vi "MGCC_FntStaMach_FSM loop.vi"() -> (0 "Function":bool[](array[boolean]), 1 "State":bool[](array[boolean]), 2 "Name of state":string[](array[string]), 3 "Name_Function":string[](array[string]), 4 "Next State":string, 5 "Current State":string)   [LabVIEW 2016]
doc: "This VI is the main loop for the FSM in MGCC. The inputs are the events while the output is the name of the next state."
uses:
  <vilib>/imath/engines/lvmath2/RunTimeEngine/IndexRead/NIMS V(S).vi
  <instcachedir>/0/NIMS V(S)_0488751826AF41519A22953C041130DC.lvgen/NIMS V(S)_0488751826AF41519A22953C041130DC_003.vi
  <vilib>/imathl/engines/lvmath/Functions/Error Handling/Create Error.vi
  <vilib>/imath/engines/lvmath2/RunTimeEngine/NodeEndStatement/NIMS_NodeEndStatement_Output.vi
  <instcachedir>/0/NIMS_NodeEndStatement_Output_53EC0D466D134D7ABD903AC30B43404B.lvgen/NIMS_NodeEndStatement_Output_53EC0D466D134D7ABD903AC30B43404B_011.vi
  <vilib>/imath/engines/lvmath2/RunTimeEngine/ErrorHandling/NIMS_Finalize Error.vi
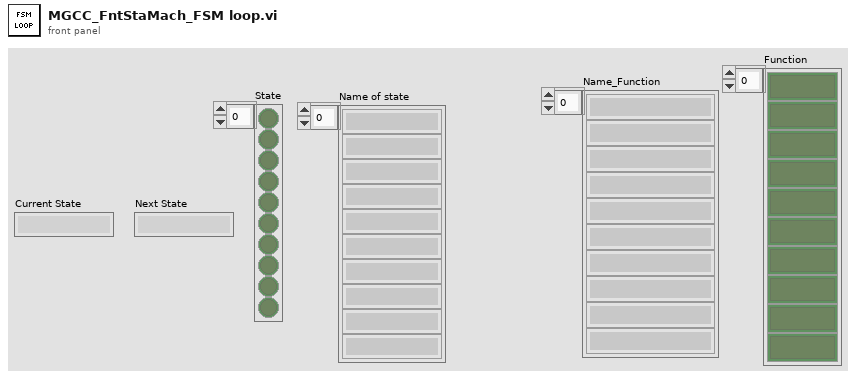
[diagram p1: front panel]
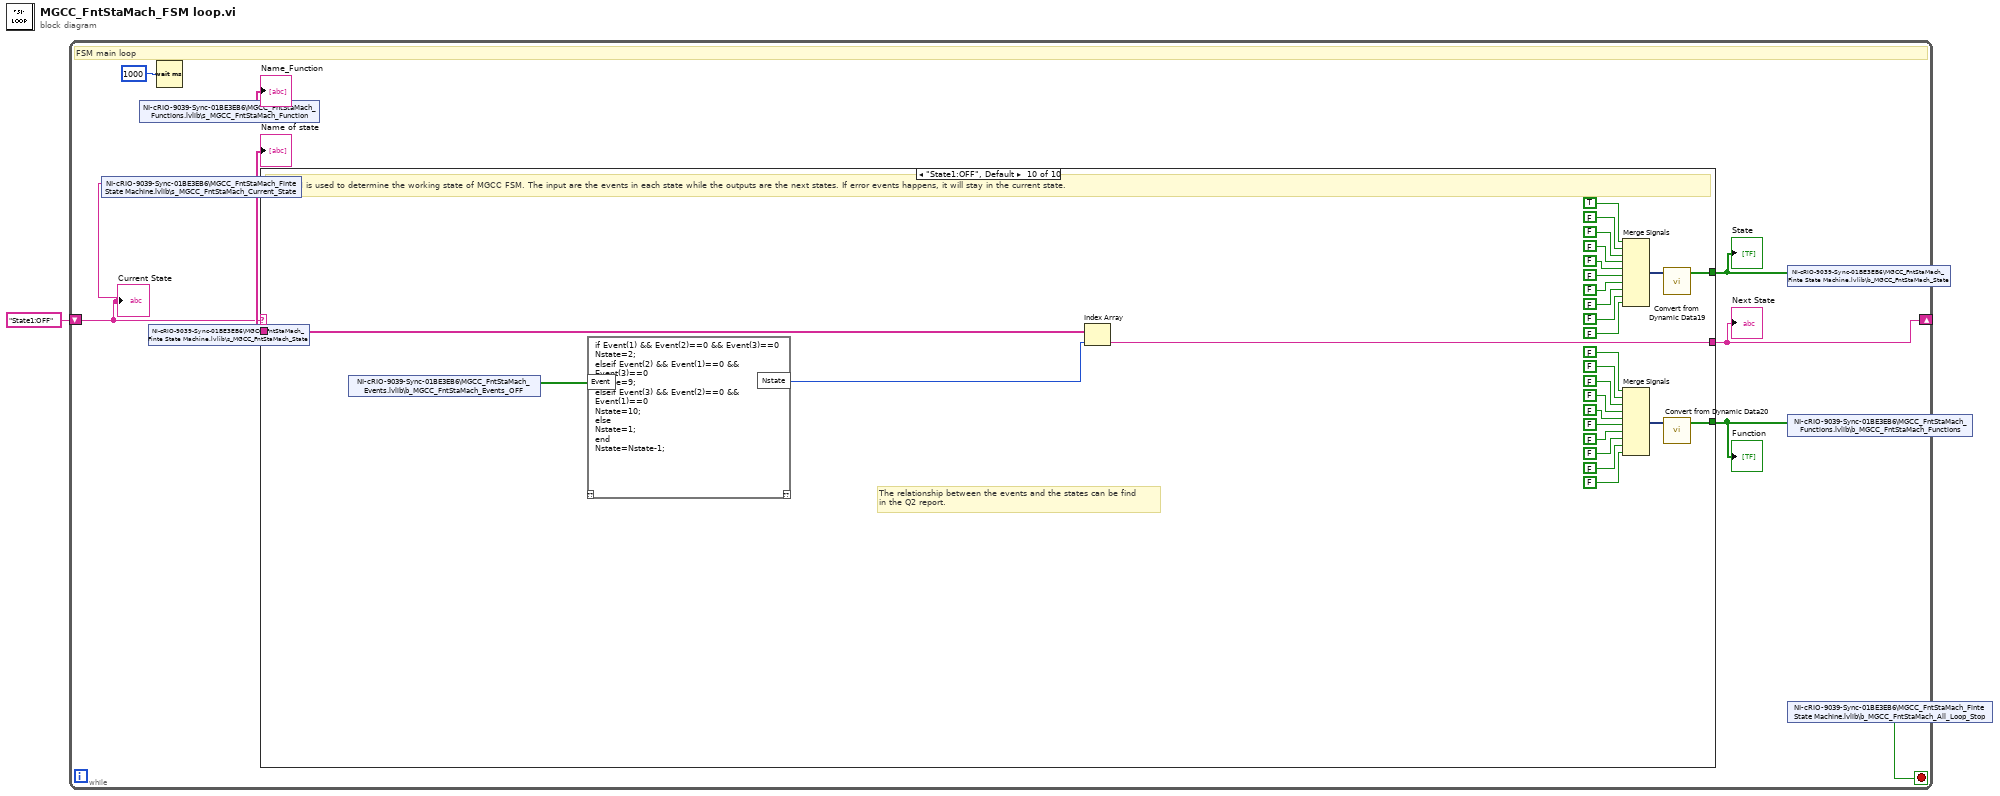
[diagram p0: block diagram]
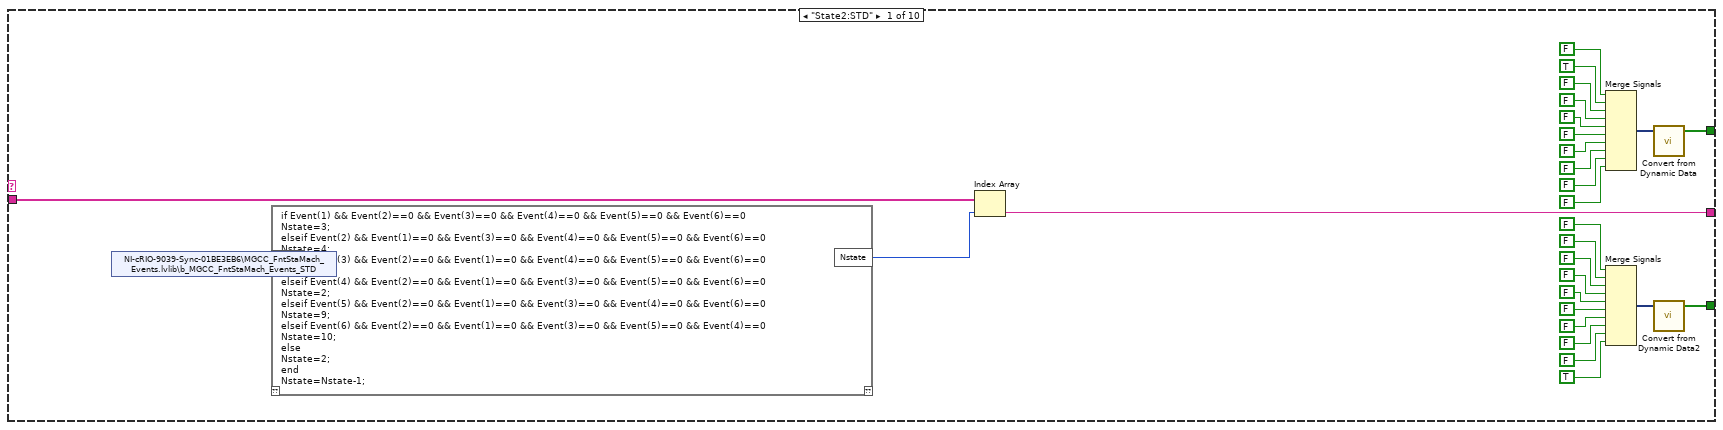
[diagram p2: hidden frame]
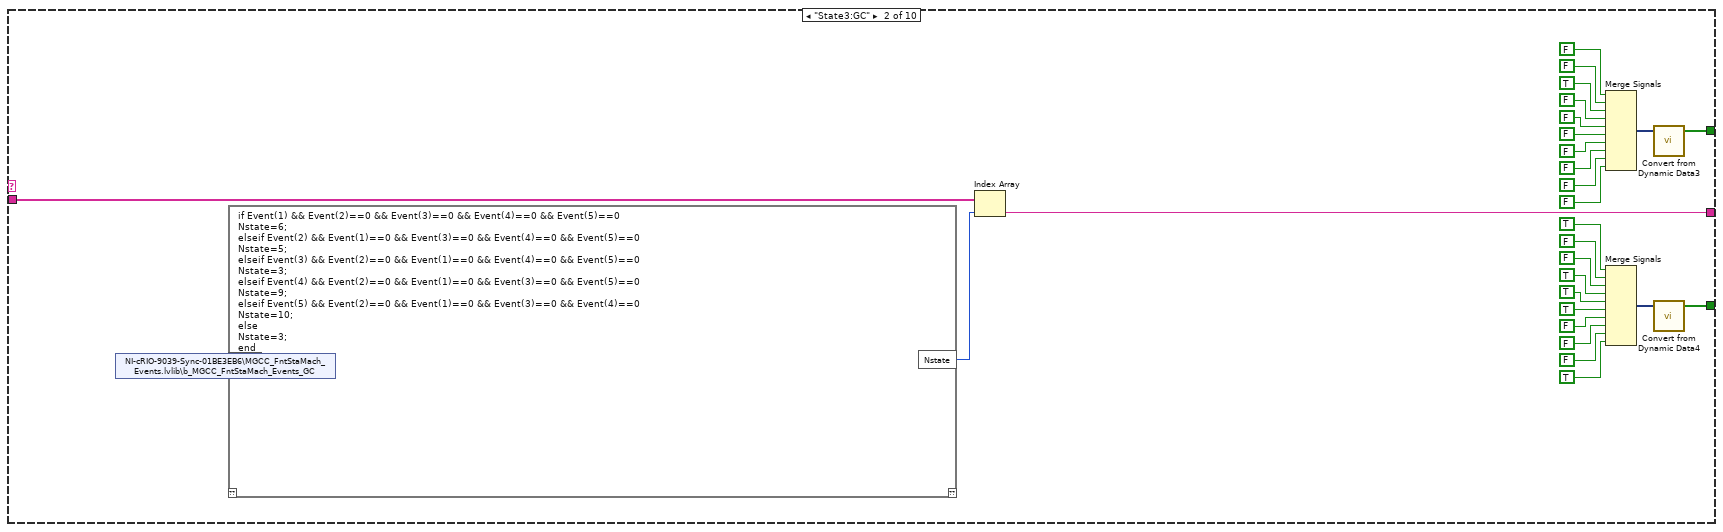
[diagram p3: hidden frame]
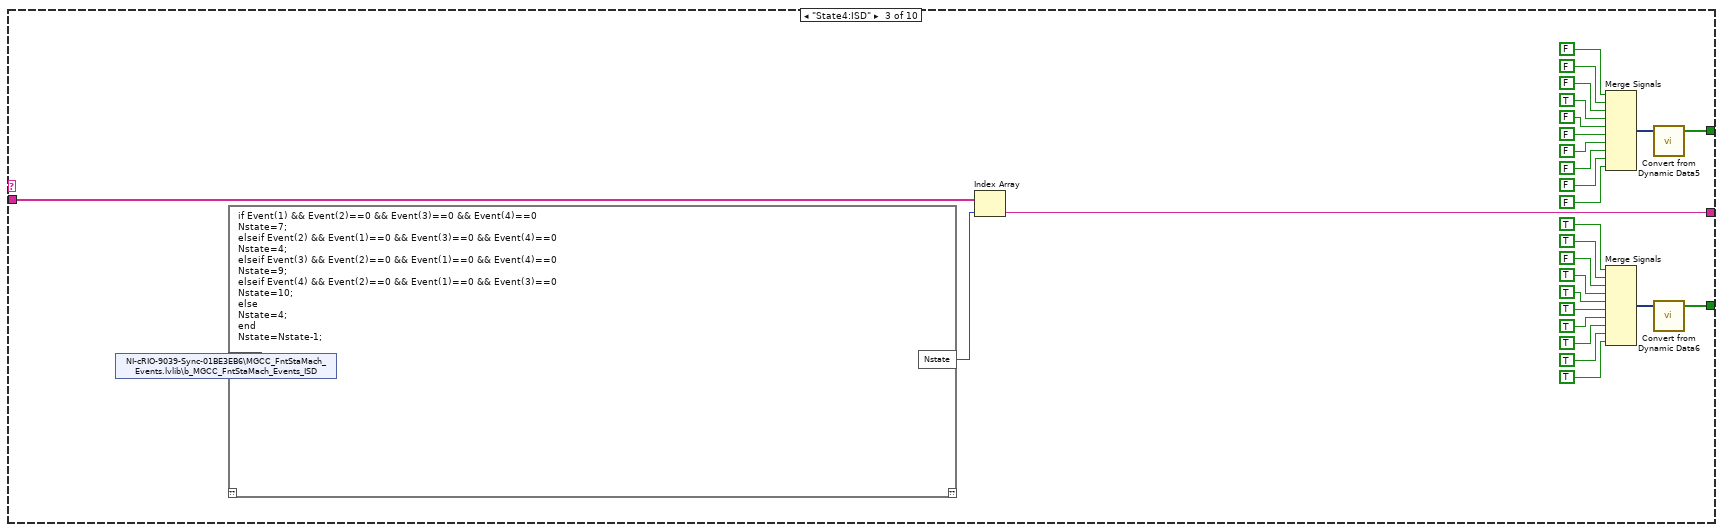
[diagram p4: hidden frame]
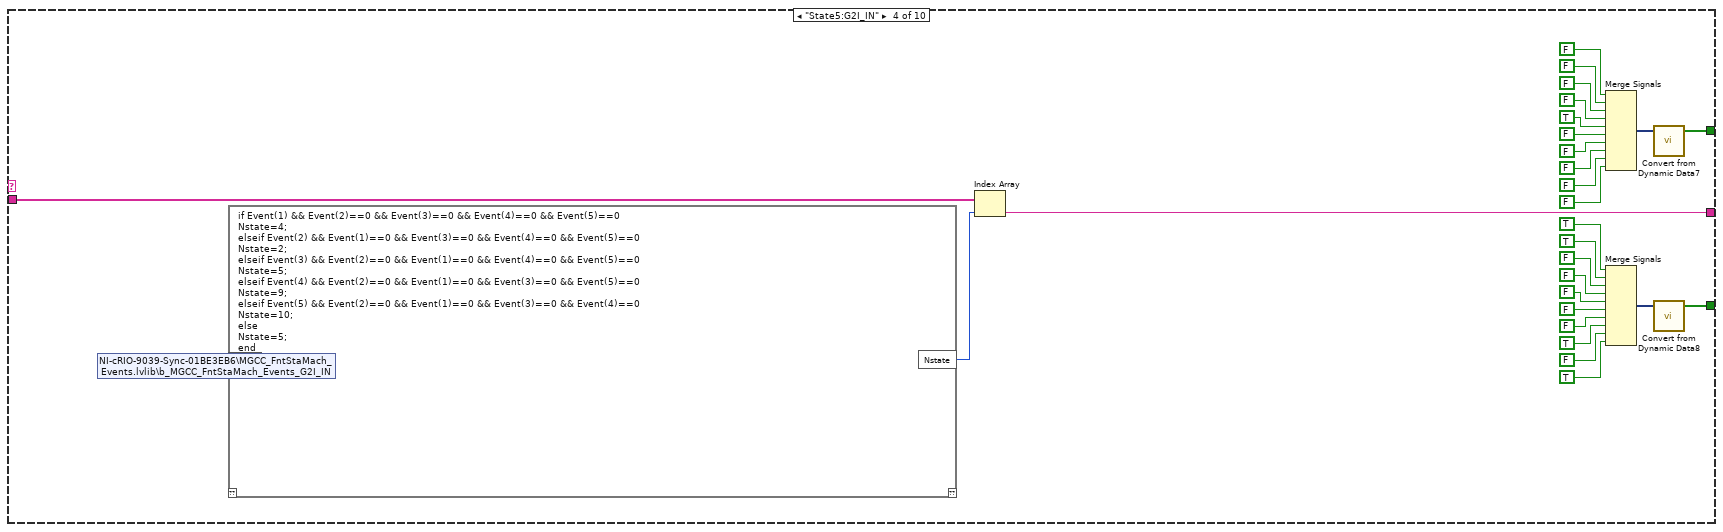
[diagram p5: hidden frame]
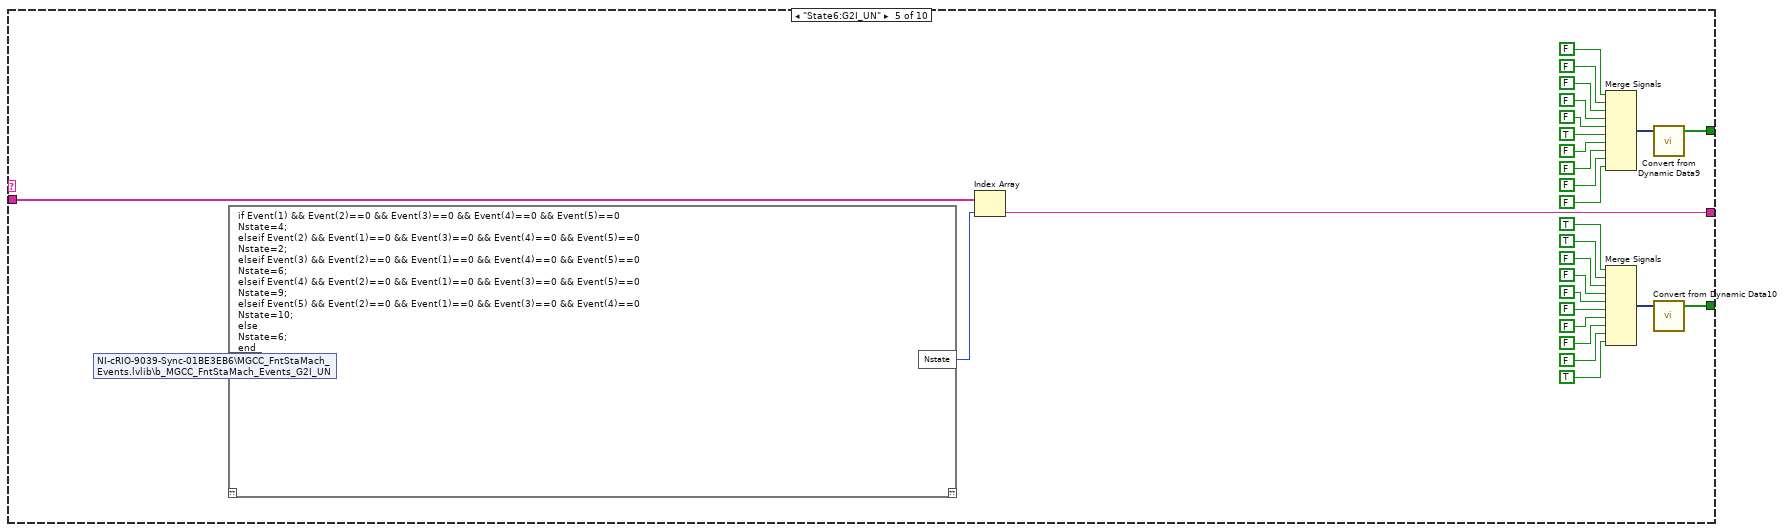
[diagram p6: hidden frame]
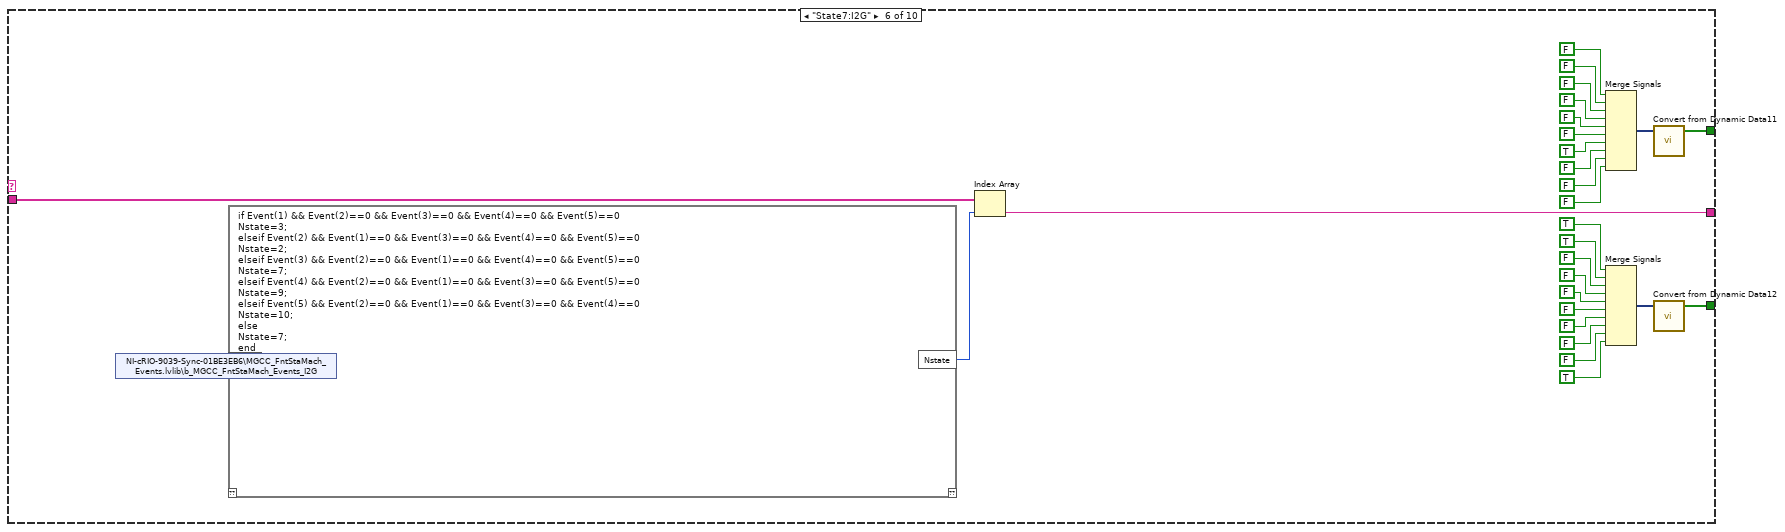
[diagram p7: hidden frame]
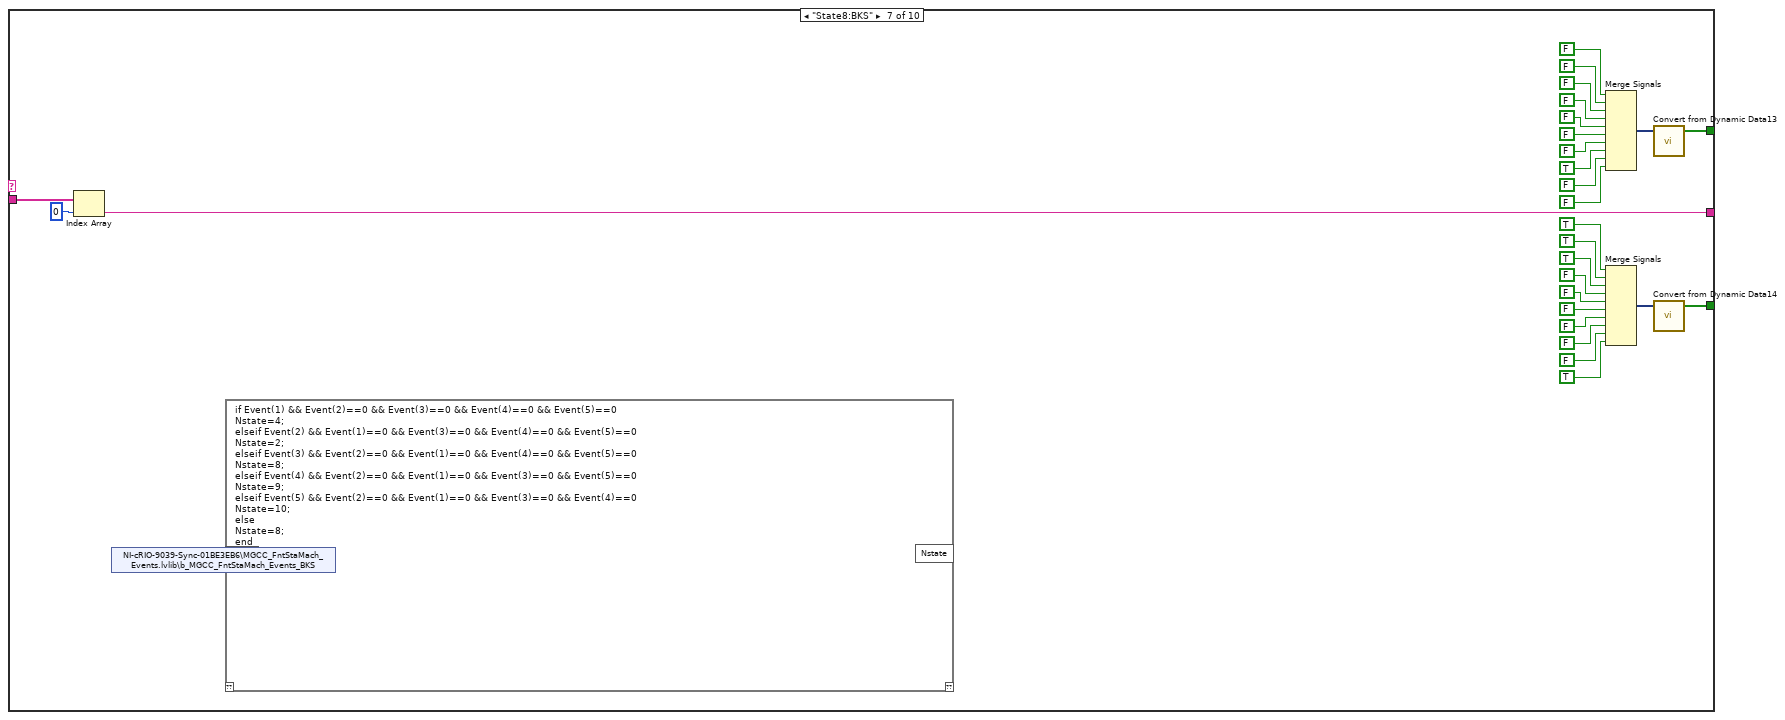
[diagram p8: hidden frame]
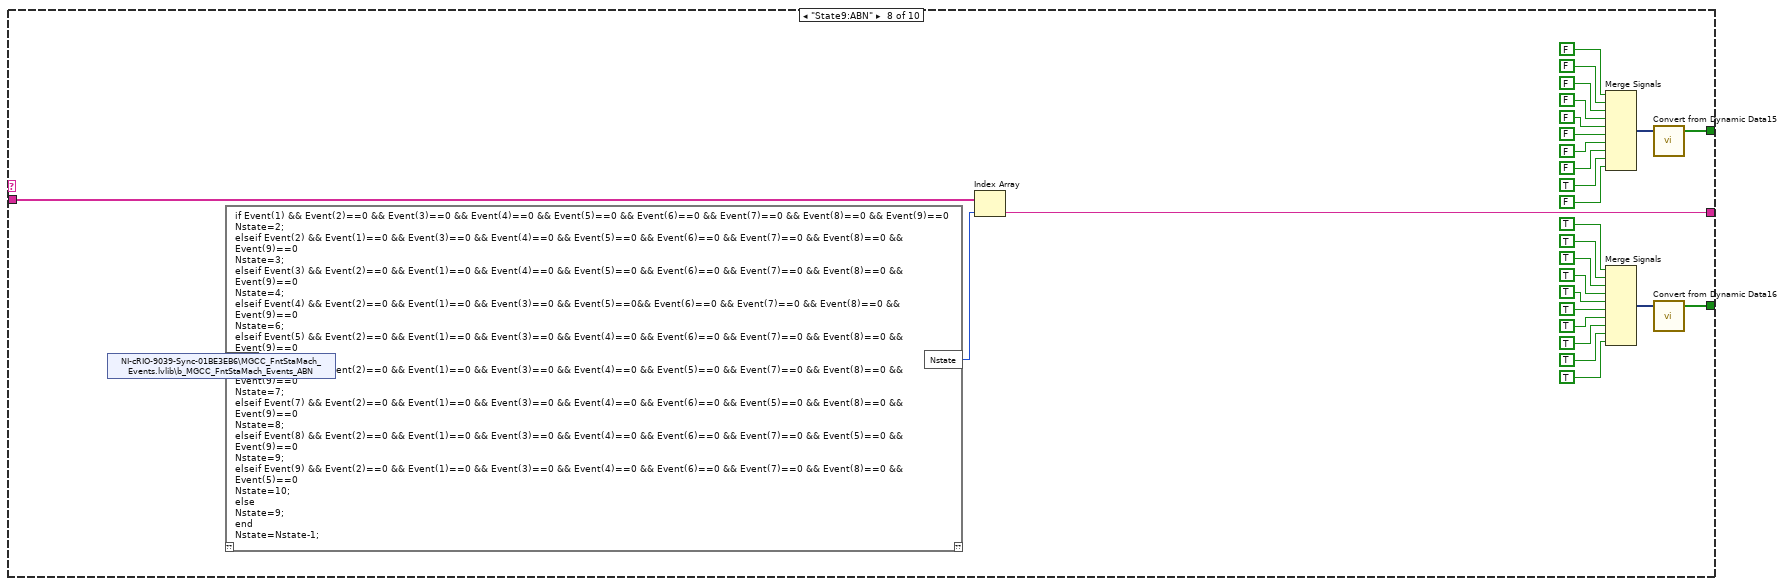
[diagram p9: hidden frame]
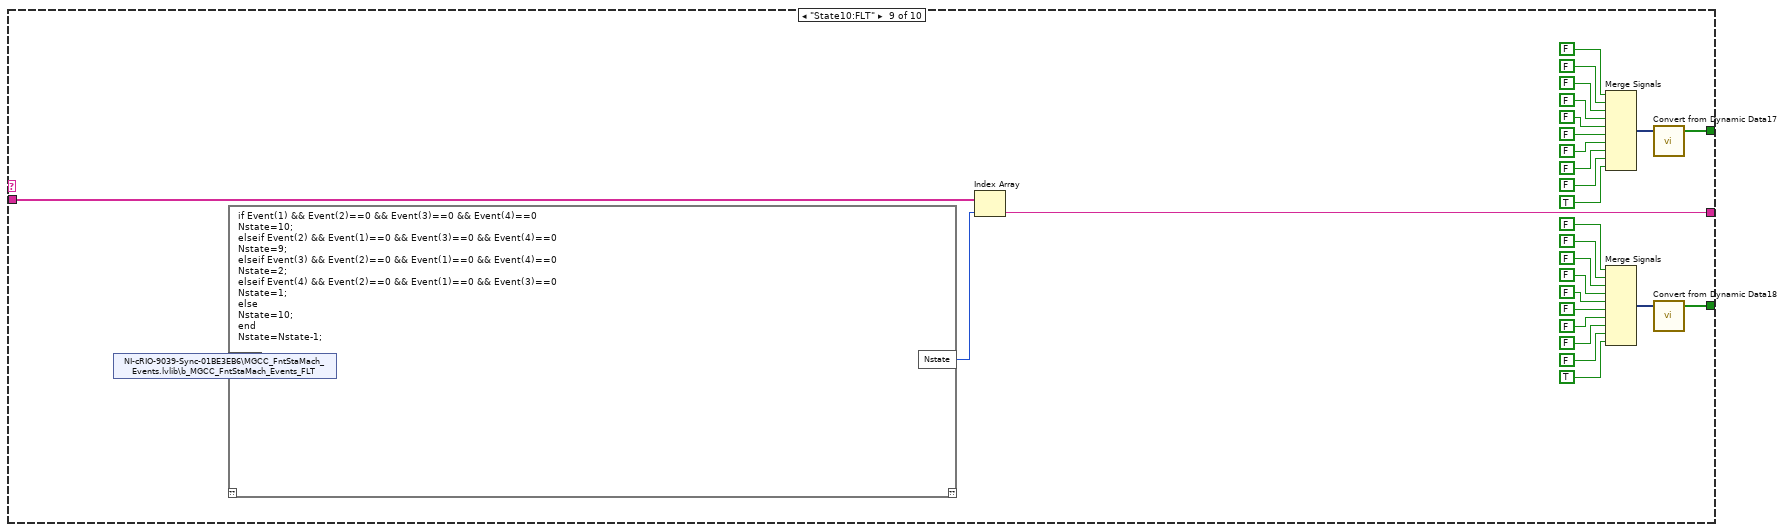
[diagram p10: hidden frame]
diagram:
  n1 = while {
    shift-right: [w9] -> _
    shift-left: "State1:OFF" ("String") -> [w2]
    stop <- w3 stop-if-true
    # "FSM main loop"
    n2 = shared-variable "NI-cRIO-9039-Sync-01BE3EB6\\MGCC_FntStaMach_Finte State Machine.lvlib\\s_MGCC_FntStaMach_Current_State"(w2) -> ()  [unwired: 1 in, 1 out]
    n3 = shared-variable "NI-cRIO-9039-Sync-01BE3EB6\\MGCC_FntStaMach_Functions.lvlib\\s_MGCC_FntStaMach_Function"() -> (→"Name_Function":string[])  [unwired: 1 in, 1 out]
    n4 = shared-variable "NI-cRIO-9039-Sync-01BE3EB6\\MGCC_FntStaMach_Finte State Machine.lvlib\\s_MGCC_FntStaMach_State"() -> (w7:string[])  [unwired: 1 in, 1 out]
    "Name of state" <- w7
    n5 = Wait (ms)(milliseconds to wait=u32 1000) -> ()  [unwired: 1 out]
    n6 = case shown="\"State1:OFF\", Default" w2 {
      tunnel: [w37 w1004 w1703 w2172 w2871 w3570 w4268 w4968 w7087 w7568] -> w9
      tunnel: [w25 w1005 w1704 w2173 w2872 w3571 w4270 w4969 w7088 w7556] -> w6
      tunnel: w7 -> [w24 w1003 w1702 w2171 w2870 w3569 w4267 w4967 w7086 w7555]
      tunnel: [w10 w989 w1688 w2157 w2856 w3555 w4254 w4953 w7072 w7541] -> w5
      frame "State2:STD" {
        n7 = shared-variable "NI-cRIO-9039-Sync-01BE3EB6\\MGCC_FntStaMach_Events.lvlib\\b_MGCC_FntStaMach_Events_STD"() -> (w23:bool[])  [unwired: 1 in, 1 out]
        n8 = mathscript code="if Event(1) && Event(2)==0 && Event(3)==0 && Event(4)==0 && Event(5)==0 && Event(6)==0\nNstate=3;\nelseif Event(2) && Event(1)==0 && Event(3)==0 && Event(4)==0 && Event(5)==0 && Event(6)==0\nNstate=4;\nelseif Event(3) && Event(2)==0 && Event(1)==0 && Event(4)==0 && Event(5)==0 && Event(6)==0\nNstate=8;\nelseif Event(4) && Event(2)==0 && Event(1)==0 && Event(3)==0 && Event(5)==0 && Event(6)==0\nNstate=2;\nelseif Event(5) && Event(2)==0 && Event(1)==0 && Event(3)==0 && Event(4)==0 && Event(6)==0\nNstate=9;\nelseif Event(6) && Event(2)==0 && Event(1)==0 && Event(3)==0 && Event(5)==0 && Event(4)==0\nNstate=10;\nelse\nNstate=2;\nend\nNstate=Nstate-1;"("Event"=w23) -> ("Nstate"=w22:i32)  [unwired: 1 in, 1 out]
        n9 = Index Array(array=w24, index=w22) -> (element=w37:string)
        n10 = Merge Signals(FALSE ("State3"), TRUE ("State3"), FALSE ("State3"), FALSE ("State3"), FALSE ("State3"), FALSE ("State3"), FALSE ("State3"), FALSE ("State3"), FALSE ("State3"), FALSE ("State3")) -> (w26:dynamicdata)
        n11 = Merge Signals(FALSE ("State3"), FALSE ("State3"), FALSE ("State3"), FALSE ("State3"), FALSE ("State3"), FALSE ("State3"), FALSE ("State3"), FALSE ("State3"), FALSE ("State3"), TRUE ("State3")) -> (w11:dynamicdata)
        n12 = call "Convert from Dynamic Data"("Dynamic Data Type"=w26) -> ("Array"=w25:bool[])  [unwired: 3 in]
        n13 = call "Convert from Dynamic Data2"("Dynamic Data Type"=w11) -> ("Array"=w10:bool[])  [unwired: 3 in]
      }
      frame "State3:GC" {
        n14 = shared-variable "NI-cRIO-9039-Sync-01BE3EB6\\MGCC_FntStaMach_Events.lvlib\\b_MGCC_FntStaMach_Events_GC"() -> (w1002:bool[])  [unwired: 1 in, 1 out]
        n15 = mathscript code="if Event(1) && Event(2)==0 && Event(3)==0 && Event(4)==0 && Event(5)==0 \nNstate=6;\nelseif Event(2) && Event(1)==0 && Event(3)==0 && Event(4)==0 && Event(5)==0 \nNstate=5;\nelseif Event(3) && Event(2)==0 && Event(1)==0 && Event(4)==0 && Event(5)==0 \nNstate=3;\nelseif Event(4) && Event(2)==0 && Event(1)==0 && Event(3)==0 && Event(5)==0\nNstate=9;\nelseif Event(5) && Event(2)==0 && Event(1)==0 && Event(3)==0 && Event(4)==0 \nNstate=10;\nelse\nNstate=3;\nend\nNstate=Nstate-1;"("Event"=w1002) -> ("Nstate"=w1001:i32)  [unwired: 1 in, 1 out]
        n16 = Index Array(array=w1003, index=w1001) -> (element=w1004:string)
        n17 = Merge Signals(FALSE ("State3"), FALSE ("State3"), TRUE ("State3"), FALSE ("State3"), FALSE ("State3"), FALSE ("State3"), FALSE ("State3"), FALSE ("State3"), FALSE ("State3"), FALSE ("State3")) -> (w1006:dynamicdata)
        n18 = Merge Signals(TRUE ("State3"), FALSE ("State3"), FALSE ("State3"), TRUE ("State3"), TRUE ("State3"), TRUE ("State3"), FALSE ("State3"), FALSE ("State3"), FALSE ("State3"), TRUE ("State3")) -> (w990:dynamicdata)
        n19 = call "Convert from Dynamic Data3"("Dynamic Data Type"=w1006) -> ("Array"=w1005:bool[])  [unwired: 3 in]
        n20 = call "Convert from Dynamic Data4"("Dynamic Data Type"=w990) -> ("Array"=w989:bool[])  [unwired: 3 in]
      }
      frame "State4:ISD" {
        n21 = shared-variable "NI-cRIO-9039-Sync-01BE3EB6\\MGCC_FntStaMach_Events.lvlib\\b_MGCC_FntStaMach_Events_ISD"() -> (w1701:bool[])  [unwired: 1 in, 1 out]
        n22 = mathscript code="if Event(1) && Event(2)==0 && Event(3)==0 && Event(4)==0 \nNstate=7;\nelseif Event(2) && Event(1)==0 && Event(3)==0 && Event(4)==0 \nNstate=4;\nelseif Event(3) && Event(2)==0 && Event(1)==0 && Event(4)==0 \nNstate=9;\nelseif Event(4) && Event(2)==0 && Event(1)==0 && Event(3)==0 \nNstate=10;\nelse\nNstate=4;\nend\nNstate=Nstate-1;"("Event"=w1701) -> ("Nstate"=w1700:i32)  [unwired: 1 in, 1 out]
        n23 = Index Array(array=w1702, index=w1700) -> (element=w1703:string)
        n24 = Merge Signals(FALSE ("State3"), FALSE ("State3"), FALSE ("State3"), TRUE ("State3"), FALSE ("State3"), FALSE ("State3"), FALSE ("State3"), FALSE ("State3"), FALSE ("State3"), FALSE ("State3")) -> (w1705:dynamicdata)
        n25 = Merge Signals(TRUE ("State3"), TRUE ("State3"), FALSE ("State3"), TRUE ("State3"), TRUE ("State3"), TRUE ("State3"), TRUE ("State3"), TRUE ("State3"), TRUE ("State3"), TRUE ("State3")) -> (w1689:dynamicdata)
        n26 = call "Convert from Dynamic Data5"("Dynamic Data Type"=w1705) -> ("Array"=w1704:bool[])  [unwired: 3 in]
        n27 = call "Convert from Dynamic Data6"("Dynamic Data Type"=w1689) -> ("Array"=w1688:bool[])  [unwired: 3 in]
      }
      frame "State5:G2I_IN" {
        n28 = shared-variable "NI-cRIO-9039-Sync-01BE3EB6\\MGCC_FntStaMach_Events.lvlib\\b_MGCC_FntStaMach_Events_G2I_IN"() -> (w2170:bool[])  [unwired: 1 in, 1 out]
        n29 = mathscript code="if Event(1) && Event(2)==0 && Event(3)==0 && Event(4)==0 && Event(5)==0 \nNstate=4;\nelseif Event(2) && Event(1)==0 && Event(3)==0 && Event(4)==0 && Event(5)==0 \nNstate=2;\nelseif Event(3) && Event(2)==0 && Event(1)==0 && Event(4)==0 && Event(5)==0 \nNstate=5;\nelseif Event(4) && Event(2)==0 && Event(1)==0 && Event(3)==0 && Event(5)==0\nNstate=9;\nelseif Event(5) && Event(2)==0 && Event(1)==0 && Event(3)==0 && Event(4)==0 \nNstate=10;\nelse\nNstate=5;\nend\nNstate=Nstate-1;"("Event"=w2170) -> ("Nstate"=w2169:i32)  [unwired: 1 in, 1 out]
        n30 = Index Array(array=w2171, index=w2169) -> (element=w2172:string)
        n31 = Merge Signals(FALSE ("State3"), FALSE ("State3"), FALSE ("State3"), FALSE ("State3"), TRUE ("State3"), FALSE ("State3"), FALSE ("State3"), FALSE ("State3"), FALSE ("State3"), FALSE ("State3")) -> (w2174:dynamicdata)
        n32 = Merge Signals(TRUE ("State3"), TRUE ("State3"), FALSE ("State3"), FALSE ("State3"), FALSE ("State3"), FALSE ("State3"), FALSE ("State3"), TRUE ("State3"), FALSE ("State3"), TRUE ("State3")) -> (w2158:dynamicdata)
        n33 = call "Convert from Dynamic Data7"("Dynamic Data Type"=w2174) -> ("Array"=w2173:bool[])  [unwired: 3 in]
        n34 = call "Convert from Dynamic Data8"("Dynamic Data Type"=w2158) -> ("Array"=w2157:bool[])  [unwired: 3 in]
      }
      frame "State6:G2I_UN" {
        n35 = shared-variable "NI-cRIO-9039-Sync-01BE3EB6\\MGCC_FntStaMach_Events.lvlib\\b_MGCC_FntStaMach_Events_G2I_UN"() -> (w2868:bool[])  [unwired: 1 in, 1 out]
        n36 = mathscript code="if Event(1) && Event(2)==0 && Event(3)==0 && Event(4)==0 && Event(5)==0 \nNstate=4;\nelseif Event(2) && Event(1)==0 && Event(3)==0 && Event(4)==0 && Event(5)==0 \nNstate=2;\nelseif Event(3) && Event(2)==0 && Event(1)==0 && Event(4)==0 && Event(5)==0 \nNstate=6;\nelseif Event(4) && Event(2)==0 && Event(1)==0 && Event(3)==0 && Event(5)==0\nNstate=9;\nelseif Event(5) && Event(2)==0 && Event(1)==0 && Event(3)==0 && Event(4)==0 \nNstate=10;\nelse\nNstate=6;\nend\nNstate=Nstate-1;"("Event"=w2868) -> ("Nstate"=w2869:i32)  [unwired: 1 in, 1 out]
        n37 = Index Array(array=w2870, index=w2869) -> (element=w2871:string)
        n38 = Merge Signals(FALSE ("State3"), FALSE ("State3"), FALSE ("State3"), FALSE ("State3"), FALSE ("State3"), TRUE ("State3"), FALSE ("State3"), FALSE ("State3"), FALSE ("State3"), FALSE ("State3")) -> (w2873:dynamicdata)
        n39 = Merge Signals(TRUE ("State3"), TRUE ("State3"), FALSE ("State3"), FALSE ("State3"), FALSE ("State3"), FALSE ("State3"), FALSE ("State3"), FALSE ("State3"), FALSE ("State3"), TRUE ("State3")) -> (w2857:dynamicdata)
        n40 = call "Convert from Dynamic Data9"("Dynamic Data Type"=w2873) -> ("Array"=w2872:bool[])  [unwired: 3 in]
        n41 = call "Convert from Dynamic Data10"("Dynamic Data Type"=w2857) -> ("Array"=w2856:bool[])  [unwired: 3 in]
      }
      frame "State7:I2G" {
        n42 = shared-variable "NI-cRIO-9039-Sync-01BE3EB6\\MGCC_FntStaMach_Events.lvlib\\b_MGCC_FntStaMach_Events_I2G"() -> (w3567:bool[])  [unwired: 1 in, 1 out]
        n43 = mathscript code="if Event(1) && Event(2)==0 && Event(3)==0 && Event(4)==0 && Event(5)==0 \nNstate=3;\nelseif Event(2) && Event(1)==0 && Event(3)==0 && Event(4)==0 && Event(5)==0 \nNstate=2;\nelseif Event(3) && Event(2)==0 && Event(1)==0 && Event(4)==0 && Event(5)==0 \nNstate=7;\nelseif Event(4) && Event(2)==0 && Event(1)==0 && Event(3)==0 && Event(5)==0\nNstate=9;\nelseif Event(5) && Event(2)==0 && Event(1)==0 && Event(3)==0 && Event(4)==0 \nNstate=10;\nelse\nNstate=7;\nend\nNstate=Nstate-1;"("Event"=w3567) -> ("Nstate"=w3568:i32)  [unwired: 1 in, 1 out]
        n44 = Index Array(array=w3569, index=w3568) -> (element=w3570:string)
        n45 = Merge Signals(FALSE ("State3"), FALSE ("State3"), FALSE ("State3"), FALSE ("State3"), FALSE ("State3"), FALSE ("State3"), TRUE ("State3"), FALSE ("State3"), FALSE ("State3"), FALSE ("State3")) -> (w3572:dynamicdata)
        n46 = Merge Signals(TRUE ("State3"), TRUE ("State3"), FALSE ("State3"), FALSE ("State3"), FALSE ("State3"), FALSE ("State3"), FALSE ("State3"), FALSE ("State3"), FALSE ("State3"), TRUE ("State3")) -> (w3556:dynamicdata)
        n47 = call "Convert from Dynamic Data11"("Dynamic Data Type"=w3572) -> ("Array"=w3571:bool[])  [unwired: 3 in]
        n48 = call "Convert from Dynamic Data12"("Dynamic Data Type"=w3556) -> ("Array"=w3555:bool[])  [unwired: 3 in]
      }
      frame "State8:BKS" {
        n49 = Index Array(array=w4267, index=0) -> (element=w4268:string)
        n50 = shared-variable "NI-cRIO-9039-Sync-01BE3EB6\\MGCC_FntStaMach_Events.lvlib\\b_MGCC_FntStaMach_Events_BKS"() -> (w4266:bool[])  [unwired: 1 in, 1 out]
        n51 = mathscript code="if Event(1) && Event(2)==0 && Event(3)==0 && Event(4)==0 && Event(5)==0 \nNstate=4;\nelseif Event(2) && Event(1)==0 && Event(3)==0 && Event(4)==0 && Event(5)==0 \nNstate=2;\nelseif Event(3) && Event(2)==0 && Event(1)==0 && Event(4)==0 && Event(5)==0 \nNstate=8;\nelseif Event(4) && Event(2)==0 && Event(1)==0 && Event(3)==0 && Event(5)==0\nNstate=9;\nelseif Event(5) && Event(2)==0 && Event(1)==0 && Event(3)==0 && Event(4)==0 \nNstate=10;\nelse\nNstate=8;\nend\nNstate=Nstate-1;"("Event"=w4266) -> ()  [unwired: 1 in, 2 out]
        n52 = Merge Signals(FALSE ("State3"), FALSE ("State3"), FALSE ("State3"), FALSE ("State3"), FALSE ("State3"), FALSE ("State3"), FALSE ("State3"), TRUE ("State3"), FALSE ("State3"), FALSE ("State3")) -> (w4271:dynamicdata)
        n53 = Merge Signals(TRUE ("State3"), TRUE ("State3"), TRUE ("State3"), FALSE ("State3"), FALSE ("State3"), FALSE ("State3"), FALSE ("State3"), FALSE ("State3"), FALSE ("State3"), TRUE ("State3")) -> (w4255:dynamicdata)
        n54 = call "Convert from Dynamic Data13"("Dynamic Data Type"=w4271) -> ("Array"=w4270:bool[])  [unwired: 3 in]
        n55 = call "Convert from Dynamic Data14"("Dynamic Data Type"=w4255) -> ("Array"=w4254:bool[])  [unwired: 3 in]
      }
      frame "State9:ABN" {
        n56 = shared-variable "NI-cRIO-9039-Sync-01BE3EB6\\MGCC_FntStaMach_Events.lvlib\\b_MGCC_FntStaMach_Events_ABN"() -> (w4966:bool[])  [unwired: 1 in, 1 out]
        n57 = mathscript code="if Event(1) && Event(2)==0 && Event(3)==0 && Event(4)==0 && Event(5)==0 && Event(6)==0 && Event(7)==0 && Event(8)==0 && Event(9)==0 \nNstate=2;\nelseif Event(2) && Event(1)==0 && Event(3)==0 && Event(4)==0 && Event(5)==0 && Event(6)==0 && Event(7)==0 && Event(8)==0 && Event(9)==0 \nNstate=3;\nelseif Event(3) && Event(2)==0 && Event(1)==0 && Event(4)==0 && Event(5)==0 && Event(6)==0 && Event(7)==0 && Event(8)==0 && Event(9)==0 \nNstate=4;\nelseif Event(4) && Event(2)==0 && Event(1)==0 && Event(3)==0 && Event(5)==0&& Event(6)==0 && Event(7)==0 && Event(8)==0 && Event(9)==0 \nNstate=6;\nelseif Event(5) && Event(2)==0 && Event(1)==0 && Event(3)==0 && Event(4)==0 && Event(6)==0 && Event(7)==0 && Event(8)==0 && Event(9)==0 \nNstate=5;\nelseif Event(6) && Event(2)==0 && Event(1)==0 && Event(3)==0 && Event(4)==0 && Event(5)==0 && Event(7)==0 && Event(8)==0 && Event(9)==0 \nNstate=7;\nelseif Event(7) && Event(2)==0 && Event(1)==0 && Event(3)==0 && Event(4)==0 && Event(6)==0 && Event(5)==0 && Event(8)==0 && Event(9)==0 \nNstate=8;\nelseif Event(8) && Event(2)==0 && Event(1)==0 && Event(3)==0 && Event(4)==0 && Event(6)==0 && Event(7)==0 && Event(5)==0 && Event(9)==0 \nNstate=9;\nelseif Event(9) && Event(2)==0 && Event(1)==0 && Event(3)==0 && Event(4)==0 && Event(6)==0 && Event(7)==0 && Event(8)==0 && Event(5)==0 \nNstate=10;\nelse\nNstate=9;\nend\nNstate=Nstate-1;"("Event"=w4966) -> ("Nstate"=w4965:i32)  [unwired: 1 in, 1 out]
        n58 = Index Array(array=w4967, index=w4965) -> (element=w4968:string)
        n59 = Merge Signals(FALSE ("State3"), FALSE ("State3"), FALSE ("State3"), FALSE ("State3"), FALSE ("State3"), FALSE ("State3"), FALSE ("State3"), FALSE ("State3"), TRUE ("State3"), FALSE ("State3")) -> (w4970:dynamicdata)
        n60 = Merge Signals(TRUE ("State3"), TRUE ("State3"), TRUE ("State3"), TRUE ("State3"), TRUE ("State3"), TRUE ("State3"), TRUE ("State3"), TRUE ("State3"), TRUE ("State3"), TRUE ("State3")) -> (w4954:dynamicdata)
        n61 = call "Convert from Dynamic Data15"("Dynamic Data Type"=w4970) -> ("Array"=w4969:bool[])  [unwired: 3 in]
        n62 = call "Convert from Dynamic Data16"("Dynamic Data Type"=w4954) -> ("Array"=w4953:bool[])  [unwired: 3 in]
      }
      frame "State10:FLT" {
        n63 = shared-variable "NI-cRIO-9039-Sync-01BE3EB6\\MGCC_FntStaMach_Events.lvlib\\b_MGCC_FntStaMach_Events_FLT"() -> (w7085:bool[])  [unwired: 1 in, 1 out]
        n64 = mathscript code="if Event(1) && Event(2)==0 && Event(3)==0 && Event(4)==0 \nNstate=10;\nelseif Event(2) && Event(1)==0 && Event(3)==0 && Event(4)==0 \nNstate=9;\nelseif Event(3) && Event(2)==0 && Event(1)==0 && Event(4)==0 \nNstate=2;\nelseif Event(4) && Event(2)==0 && Event(1)==0 && Event(3)==0 \nNstate=1;\nelse\nNstate=10;\nend\nNstate=Nstate-1;"("Event"=w7085) -> ("Nstate"=w7084:i32)  [unwired: 1 in, 1 out]
        n65 = Index Array(array=w7086, index=w7084) -> (element=w7087:string)
        n66 = Merge Signals(FALSE ("State3"), FALSE ("State3"), FALSE ("State3"), FALSE ("State3"), FALSE ("State3"), FALSE ("State3"), FALSE ("State3"), FALSE ("State3"), FALSE ("State3"), TRUE ("State3")) -> (w7089:dynamicdata)
        n67 = Merge Signals(FALSE ("State3"), FALSE ("State3"), FALSE ("State3"), FALSE ("State3"), FALSE ("State3"), FALSE ("State3"), FALSE ("State3"), FALSE ("State3"), FALSE ("State3"), TRUE ("State3")) -> (w7073:dynamicdata)
        n68 = call "Convert from Dynamic Data17"("Dynamic Data Type"=w7089) -> ("Array"=w7088:bool[])  [unwired: 3 in]
        n69 = call "Convert from Dynamic Data18"("Dynamic Data Type"=w7073) -> ("Array"=w7072:bool[])  [unwired: 3 in]
      }
      frame "State1:OFF", Default {
        # "The relationship between the events and the states can be find\nin the Q2 report."
        # "This FSM is used to determine the working state of MGCC FSM. The input are the events in each state while the outputs are the next states. If error events happens, it will stay in the current state."
        n70 = shared-variable "NI-cRIO-9039-Sync-01BE3EB6\\MGCC_FntStaMach_Events.lvlib\\b_MGCC_FntStaMach_Events_OFF"() -> (w7554:bool[])  [unwired: 1 in, 1 out]
        n71 = mathscript code="if Event(1) && Event(2)==0 && Event(3)==0\nNstate=2;\nelseif Event(2) && Event(1)==0 && Event(3)==0\nNstate=9;\nelseif Event(3) && Event(2)==0 && Event(1)==0\nNstate=10;\nelse\nNstate=1;\nend\nNstate=Nstate-1;"("Event"=w7554) -> ("Nstate"=w7553:i32)  [unwired: 1 in, 1 out]
        n72 = Index Array(array=w7555, index=w7553) -> (element=w7568:string)
        n73 = Merge Signals(TRUE ("State3"), FALSE ("State3"), FALSE ("State3"), FALSE ("State3"), FALSE ("State3"), FALSE ("State3"), FALSE ("State3"), FALSE ("State3"), FALSE ("State3"), FALSE ("State3")) -> (w7557:dynamicdata)
        n74 = Merge Signals(FALSE ("State3"), FALSE ("State3"), FALSE ("State3"), FALSE ("State3"), FALSE ("State3"), FALSE ("State3"), FALSE ("State3"), FALSE ("State3"), FALSE ("State3"), FALSE ("State3")) -> (w7542:dynamicdata)
        n75 = call "Convert from Dynamic Data19"("Dynamic Data Type"=w7557) -> ("Array"=w7556:bool[])  [unwired: 3 in]
        n76 = call "Convert from Dynamic Data20"("Dynamic Data Type"=w7542) -> ("Array"=w7541:bool[])  [unwired: 3 in]
      }
    }
    "Next State" <- w9
    "State" <- w6
    "Function" <- w5
    n77 = shared-variable "NI-cRIO-9039-Sync-01BE3EB6\\MGCC_FntStaMach_Finte State Machine.lvlib\\b_MGCC_FntStaMach_State"(w6) -> ()  [unwired: 1 in, 1 out]
    n78 = shared-variable "NI-cRIO-9039-Sync-01BE3EB6\\MGCC_FntStaMach_Functions.lvlib\\b_MGCC_FntStaMach_Functions"(w5) -> ()  [unwired: 1 in, 1 out]
    n79 = shared-variable "NI-cRIO-9039-Sync-01BE3EB6\\MGCC_FntStaMach_Finte State Machine.lvlib\\b_MGCC_FntStaMach_All_Loop_Stop"() -> (w3:bool)  [unwired: 1 in, 1 out]
    "Current State" <- w2
  }
